vi "SR400 ResetCount.vi"(8 "error in (no error)":errorcluster, 11 "VISA Port In":refnum<visa-resource-name>="SR400") -> (0 "error out":errorcluster, 3 "VISA Port Out":refnum<visa-resource-name>="SR400")   [LabVIEW 2019]
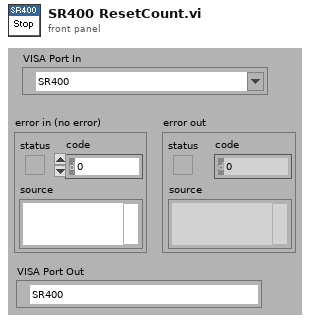
[diagram p1: front panel]
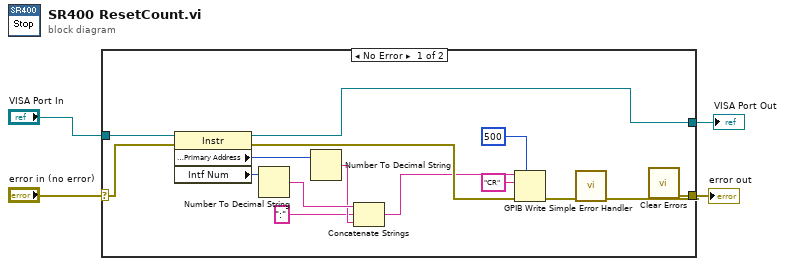
[diagram p0: block diagram]
diagram:
  n1 = case shown="No Error" "error in (no error)" {
    selector: "error in (no error)" -> [w19 w21]
    tunnel: [w9 w21] -> w3
    tunnel: "VISA Port In" -> [w18 w20]
    tunnel: [w5 w20] -> w1
    frame No Error {
      n2 = property class="Instr"(reference=w18, error in=w19) -> (reference out=w5:refnum<visa-resource-name>, error out=w17:errorcluster, "GPIB Settings:Primary Address"=w16:u16, "Intf Num"=w14:u16)
      n3 = Number To Decimal String(number=w14) -> (decimal integer string=w13:string)  [unwired: 1 in]
      n4 = Number To Decimal String(number=w16) -> (decimal integer string=w12:string)  [unwired: 1 in]
      n5 = Concatenate Strings(w13, ":" ("string"), w12) -> (w10:string)
      n6 = GPIB Write(0:w10, 1:"CR" ("data"), 3:w17, 4:500 ("timeout ms (488.2 global)")) -> (6:w15:errorcluster)  [unwired: 1 in, 1 out]
      n7 = call <vilib>:"Simple Error Handler.vi"("error in (no error)"=w15) -> ("error out"=w7:errorcluster)  [unwired: 4 in, 4 out]
      n8 = call <vilib>:"Clear Errors.vi"("error in (no error)"=w7) -> ("error out"=w9:errorcluster)  [unwired: 5 in, 1 out]
    }
    frame Error {
    }
  }
  "error out" <- w3
  "VISA Port Out" <- w1
